vi "subVI_moving avg_KA.vi"(9 "input array":dbl[](array[numeric]), 10 "sample":dbl, 11 "no. moving avg.":i32=5) -> (2 "output array":dbl[](array[numeric]), 3 "avg.":dbl)   [LabVIEW 2018]
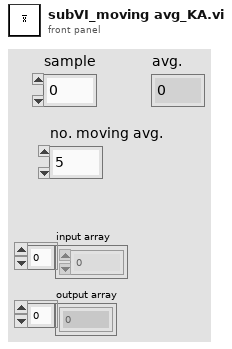
[diagram p1: front panel]
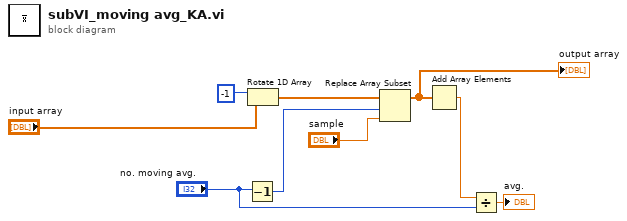
[diagram p0: block diagram]
diagram:
  n1 = Decrement(x="no. moving avg.") -> (x-1=w7:i32)
  n2 = Rotate 1D Array(1:"input array", 2:-1 ("n")) -> (0:w8:dbl[])
  n3 = Replace Array Subset(array=w8, new element="sample", index=w7) -> (w1:dbl[])
  "output array" <- w1
  n4 = Add Array Elements(numeric array=w1) -> (sum=w5:dbl)
  n5 = Divide(x=w5, y="no. moving avg.") -> (x/y=→"avg.":dbl)
